vi "Channel Write.vi"(8 "error in":errorcluster, 10 "Actuation Array":bool[](array[boolean]), 11 "DAQmx Container In":T1) -> (0 "error out":errorcluster, 2 "Actuation Array out":bool[](array[boolean]), 3 "DAQmx Container Out":T1)   [LabVIEW 2024]
uses:
  support/Control/DAQmx Container.ctl
  <vilib>/DAQmx/write.llb/DAQmx Write (Analog 1D DBL NChan 1Samp).vi
  <vilib>/DAQmx/write.llb/DAQmx Write (Digital 1D Bool NChan 1Samp 1Line).vi
  <vilib>/DAQmx/write.llb/DAQmx Write (Digital Bool 1Line 1Point).vi
  <vilib>/DAQmx/miscellaneous.llb/DAQmx Fill In Error Info.vi
panel:
  in  "Ignition Disable":bool
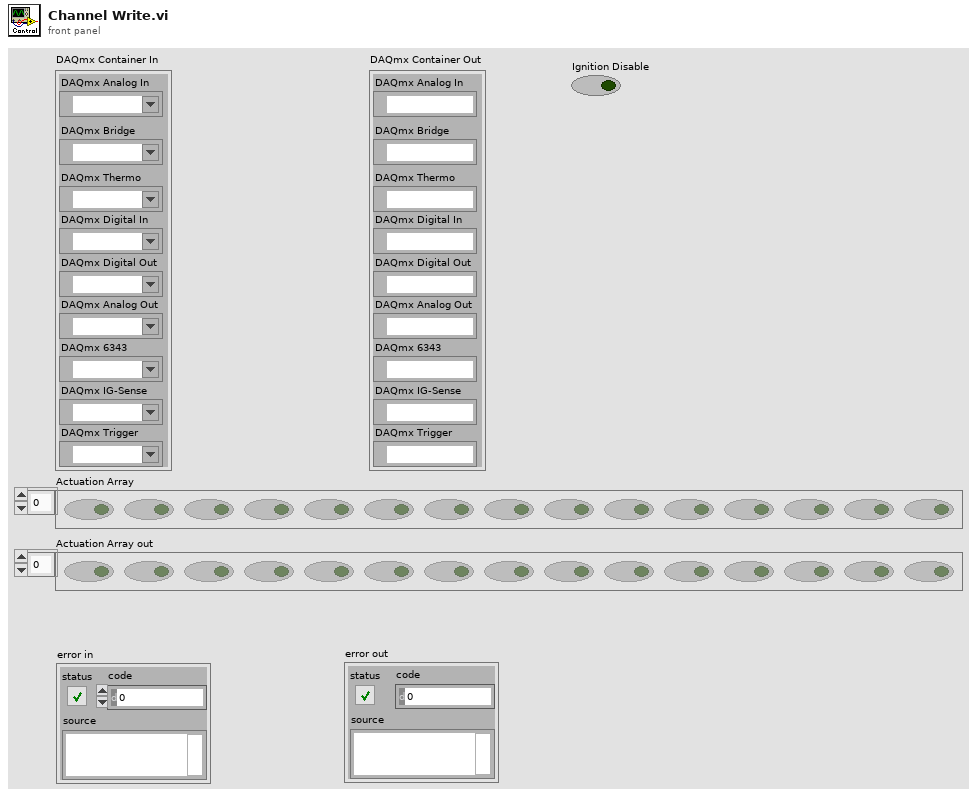
[diagram p1: front panel]
types:
  T1 = typedef "DAQmx Container.ctl" = cluster{"DAQmx Analog In":refnum<k21>, "DAQmx Digital In":refnum<k21>, "DAQmx Digital Out":refnum<k21>, "DAQmx Analog Out":refnum<k21>, "DAQmx 6343":refnum<k21>, "DAQmx IG-Sense":refnum<k21>, "DAQmx Thermo":refnum<k21>, "DAQmx Bridge":refnum<k21>, "DAQmx Trigger":refnum<k21>}
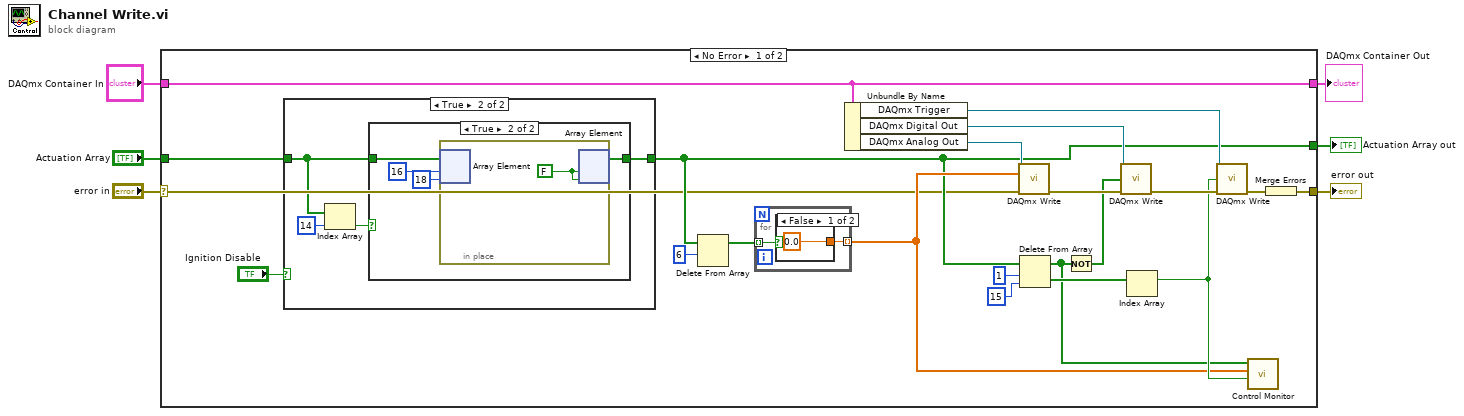
[diagram p0: block diagram]
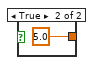
[diagram p4: hidden frame]
diagram:
  n1 = case shown="No Error" "error in" {
    selector: "error in" -> [w8 w45]
    tunnel: [w19 w45] -> w5
    tunnel: "DAQmx Container In" -> [w27 w44]
    tunnel: "Actuation Array" -> [w10 w43]
    tunnel: [w27 w44] -> w2
    tunnel: [w9 w43] -> w1
    frame No Error {
      n2 = case shown="True" "Ignition Disable" {
        tunnel: w10 -> [w28 w32]
        tunnel: [w28 w31] -> w9
        frame False {
        }
        frame True {
          n3 = Index Array(array=w32, index=14) -> (element=w29:bool)
          n4 = case shown="True" w29 {
            tunnel: w32 -> [w33 w37]
            tunnel: [w33 w36] -> w31
            frame False {
            }
            frame True {
              n5 = in-place {
                w38 = FALSE ("element")
                n6 = in-place-array #1(w37, 16, 18) -> ()  [unwired: 2 out]
                n7 = in-place-array #1(w38, w38) -> (w36:bool[])  [unwired: 2 out]
              }
            }
          }
        }
      }
      n8 = Delete From Array(array=w9, length=6) -> (array with subset deleted=w18:bool[])  [unwired: 1 in, 1 out]
      n9 = for {
        tunnel: [w40] -> w11 mode=indexing
        tunnel: w18 -> [w39] mode=indexing
        n10 = case shown="False" w39 {
          tunnel: [0.0 ("y") 5.0 ("y")] -> w40
          frame False {
          }
          frame True {
          }
        }
      }
      n11 = Unbundle By Name(w27) -> ("DAQmx Trigger"=w20:refnum<k21>, "DAQmx Digital Out"=w26:refnum<k21>, "DAQmx Analog Out"=w25:refnum<k21>)
      n12 = call-poly <vilib>:"DAQmx Write.vi"("task/channels in"=w25, "data"=w11, "error in"=w8) -> ("error out"=w24:errorcluster)  [unwired: 10 in, 2 out]
      n13 = Delete From Array(array=w9, length=1, index=15) -> (deleted portion=w16:bool[], array with subset deleted=w13:bool[])
      n14 = Not(x=w13) -> (.not. x?=w23:bool[])
      n15 = call-poly <vilib>:"DAQmx Write.vi"("task/channels in"=w26, "data"=w23, "error in"=w24) -> ("error out"=w22:errorcluster)  [unwired: 10 in, 2 out]
      n16 = Index Array(array=w16) -> (element=w14:bool)  [unwired: 1 in]
      n17 = call-poly <vilib>:"DAQmx Write.vi"("task/channels in"=w20, "data"=w14, "error in"=w22) -> ("error out"=w21:errorcluster)  [unwired: 10 in, 2 out]
      n18 = call "Control Monitor.vi"("Trigger Signal"=w14, "LED Array"=w11, "Actuation Array"=w13) -> ()  [unwired: 9 in]
      n19 = Merge Errors(w21) -> (w19:errorcluster)
    }
    frame Error {
    }
  }
  "error out" <- w5
  "DAQmx Container Out" <- w2
  "Actuation Array out" <- w1
